vi "Module Main.vi"(8 "error in (no error)":errorcluster) -> (0 "error out":errorcluster)   [LabVIEW 2026, in "Display.lvlib"]
doc: "Module Main\nFor named purposes"
uses:
  Display.lvlib
  Public Control/Elevator Direction.ctl
  Private Control/Queue FGV Action.ctl
  Error/Error.lvlib
panel:
  out "Emergency":bool
  out "Door Open":bool
  out "Elevator Direction":T1
  out "Elevator Location":dbl
  out "Timing":dbl
  # "Display Console"
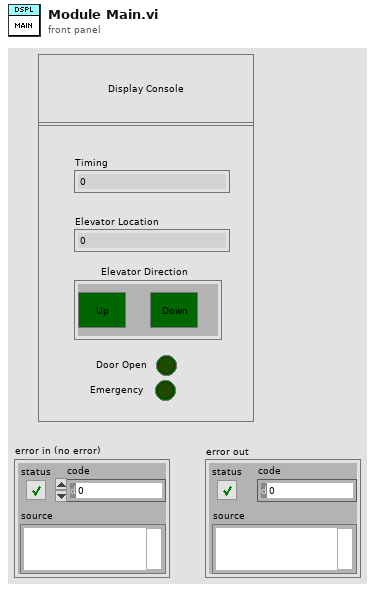
[diagram p1: front panel]
types:
  T1 = typedef "Display.lvlib/Elevator Direction.ctl" = cluster{"Up":bool, "Down":bool}
  T2 = typedef "Display.lvlib/Queue FGV Action.ctl" = enum16{"Create", "Get", "Release"}
  T3 = typedef "Display.lvlib/Queue Element.ctl" = cluster{"Module Action":T4, "Data":variant}
  T4 = typedef "Display.lvlib/Module Action.ctl" = enum16{"Init", "Error", "Exit"}
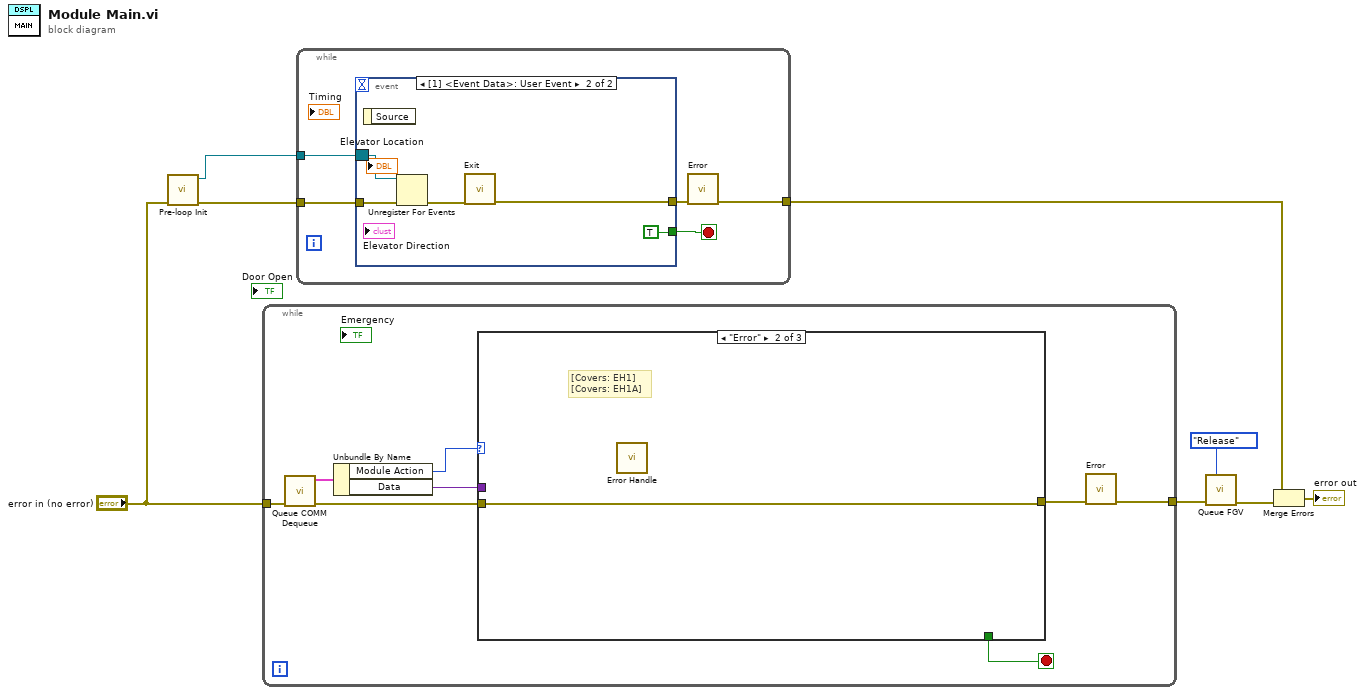
[diagram p0: block diagram]
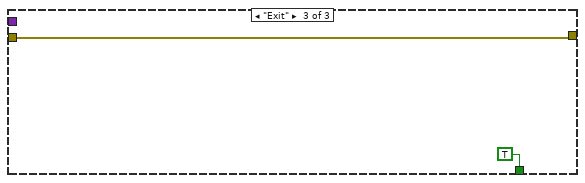
[diagram p3: hidden frame]
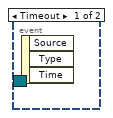
[diagram p4: hidden frame]
diagram:
  n1 = call "Pre-loop Init.vi"("error in (no error)"="error in (no error)") -> ("error out"=w7:errorcluster, "Event Registration Refnum"=w8:refnum<event-registration>)  [unwired: 9 in]
  n2 = while {
    tunnel: "error in (no error)" -> [w16]
    tunnel: [w10] -> w3
    stop <- w9 stop-if-true
    n3 = call "Queue COMM Dequeue.vi"("error in (no error)"=w16) -> ("error out"=w14:errorcluster, "element"=w15:T3)  [unwired: 9 in]
    n4 = Unbundle By Name(w15) -> ("Module Action"=w13:T4, "Data"=w12:variant)
    n5 = case shown="\"Error\"" w13 {
      tunnel: w14 -> [w17 w18 w20]
      tunnel: w12 -> [_ _ _]
      tunnel: [w17 w18 w20] -> w11
      tunnel: [_ _ TRUE] -> w9
      frame "Init", Default {
      }
      frame "Error" {
        # "[Covers: EH1] \n[Covers: EH1A]"
        n6 = call "Error Handle.vi"() -> ()  [unwired: 11 in, 1 out]
      }
      frame "Exit" {
      }
    }
    n7 = call "Error.vi"("error in (no error)"=w11) -> ("error out"=w10:errorcluster)  [unwired: 10 in]
  }
  n8 = while {
    tunnel: w8 -> [w25]
    tunnel: w7 -> [w24]
    tunnel: [w22] -> w5
    stop <- w21 stop-if-true
    n9 = event shown="[1] <Event Data>: User Event" {
      selector: w25 -> [_ w29]
      dyn-events: _ -> [_ _]
      timeout: _ -> [_ _]
      tunnel: w24 -> [_ w30]
      tunnel: [_ w27] -> w23
      tunnel: [_ TRUE] -> w21
      event Timeout {
        n10 = event-data() -> ()  [unwired: 1 in, 3 out]
      }
      event User Event {
        n11 = event-data() -> ()  [unwired: 1 in, 1 out]
        n12 = Unregister For Events(event registration refnum=w29, error in=w30) -> (error out=w28:errorcluster)
        n13 = call "Exit.vi"("error in (no error)"=w28) -> ("error out"=w27:errorcluster)  [unwired: 10 in]
      }
    }
    n14 = call "Error.vi"("error in (no error)"=w23) -> ("error out"=w22:errorcluster)  [unwired: 10 in]
  }
  n15 = call "Queue FGV.vi"("error in (no error)"=w3, "Queue FGV  Action"=Queue_FGV_Action."Release") -> ("error out"=w2:errorcluster)  [unwired: 8 in, 1 out]
  n16 = Merge Errors(w5, w2) -> (→"error out":errorcluster)
